vi "ConfigFlattenProgramToXML.vi"(8 "error in (no error)":errorcluster, 11 "ProgramArray":string[][](array[string])) -> (0 "error out":errorcluster, 3 "ProgramXML":string)   [LabVIEW 2018, in "Config.lvlib"]
uses:
  Config.lvlib
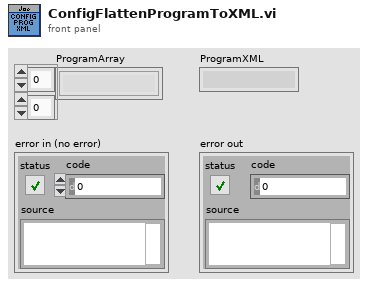
[diagram p1: front panel]
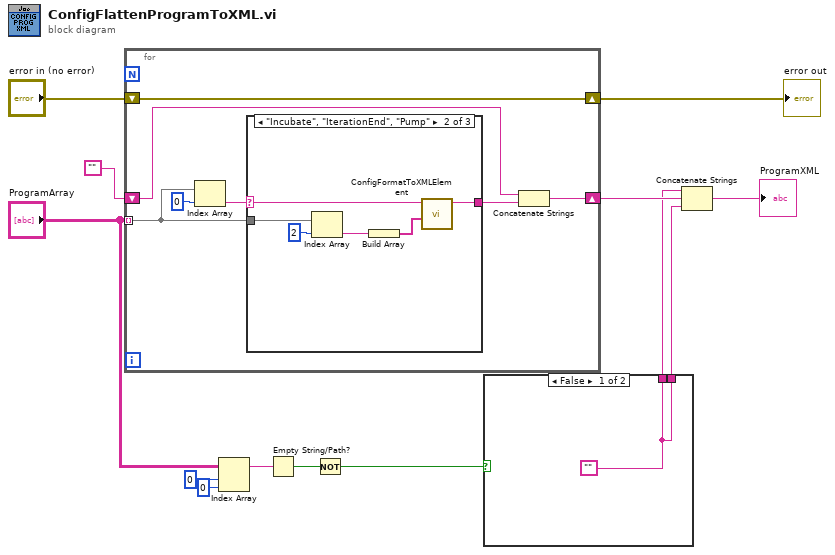
[diagram p0: block diagram]
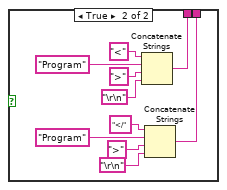
[diagram p2: hidden frame]
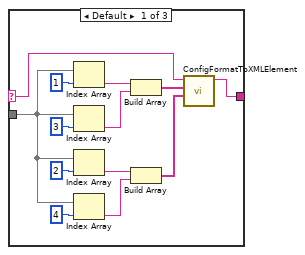
[diagram p3: hidden frame]
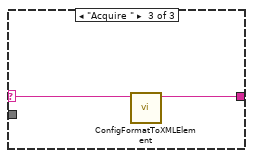
[diagram p4: hidden frame]
diagram:
  n1 = for {
    tunnel: "ProgramArray" -> [w18] mode=indexing
    shift-right: [w16] -> w10
    shift-left: "" -> [w15]
    shift-right: [w14] -> w12
    shift-left: "error in (no error)" -> [w14]
    n2 = Index Array(array=w18, index=0) -> (element=w20:string)
    n3 = case shown="\"Incubate\", \"IterationEnd\", \"Pump\"" w20 {
      selector: w20 -> [w24 w34 w40]
      tunnel: w18 -> [w22 w35 _]
      tunnel: [w21 w36 w41] -> w17
      frame Default {
        n4 = Index Array(array=w22, index=1) -> (element=w28:string)
        n5 = Index Array(array=w22, index=3) -> (element=w27:string)
        n6 = Index Array(array=w22, index=2) -> (element=w33:string)
        n7 = Index Array(array=w22, index=4) -> (element=w31:string)
        n8 = Build Array(w28, w27) -> (w23:string[])
        n9 = Build Array(w33, w31) -> (w32:string[])
        n10 = call "ConfigFormatToXMLElement.vi"("Value"=w32, "Inner Tag"=w23, "outer Tag"=w24) -> ("Resulting String"=w21:string)  [unwired: 8 in]
      }
      frame "Incubate", "IterationEnd", "Pump" {
        n11 = Index Array(array=w35, index=2) -> (element=w38:string)
        n12 = Build Array(w38) -> (w37:string[])
        n13 = call "ConfigFormatToXMLElement.vi"("Value"=w37, "outer Tag"=w34) -> ("Resulting String"=w36:string)  [unwired: 9 in]
      }
      frame "Acquire " {
        n14 = call "ConfigFormatToXMLElement.vi"("outer Tag"=w40) -> ("Resulting String"=w41:string)  [unwired: 10 in]
      }
    }
    n15 = Concatenate Strings(w15, w17) -> (w16:string)
  }
  "error out" <- w12
  n16 = Index Array(array="ProgramArray", index (row)=0 ("disabled index (row)"), index (col)=0 ("disabled index (col)")) -> (element=w4:string)
  n17 = Empty String/Path?(string/path=w4) -> (empty?=w5:bool)
  n18 = Not(x=w5) -> (.not. x?=w1:bool)
  n19 = case shown="False" w1 {
    tunnel: [w42 w51] -> w9
    tunnel: [w42 w50] -> w8
    frame False {
      w42 = ""
    }
    frame True {
      n20 = Concatenate Strings("<" ("string"), "Program" ("string"), ">" ("string"), "\r\n") -> (w50:string)
      n21 = Concatenate Strings("</" ("string"), "Program" ("string"), ">" ("string"), "\r\n") -> (w51:string)
    }
  }
  n22 = Concatenate Strings(w8, w10, w9) -> (→"ProgramXML":string)
